vi "Maps-Update.vi"(0 "Google Maps Resource In":T1, 11 "error in (no error)":errorcluster) -> (4 "Google Maps Resource Out":T1, 8 "URL":string, 15 "error out":errorcluster)   [LabVIEW 2020]
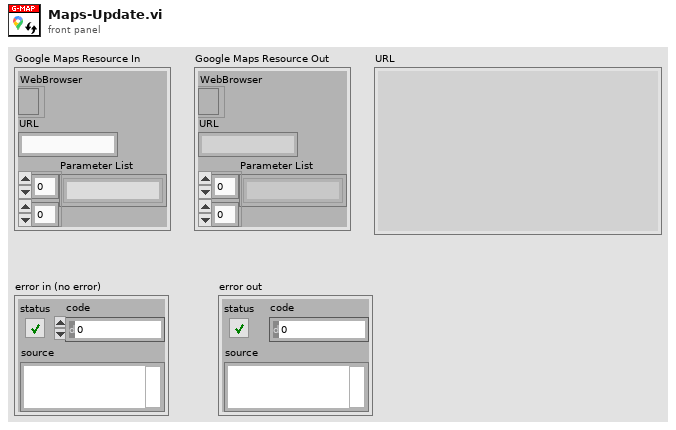
[diagram p1: front panel]
types:
  T1 = cluster{"WebBrowser":refnum<k7>, "URL":string, "Parameter List":string[][]}
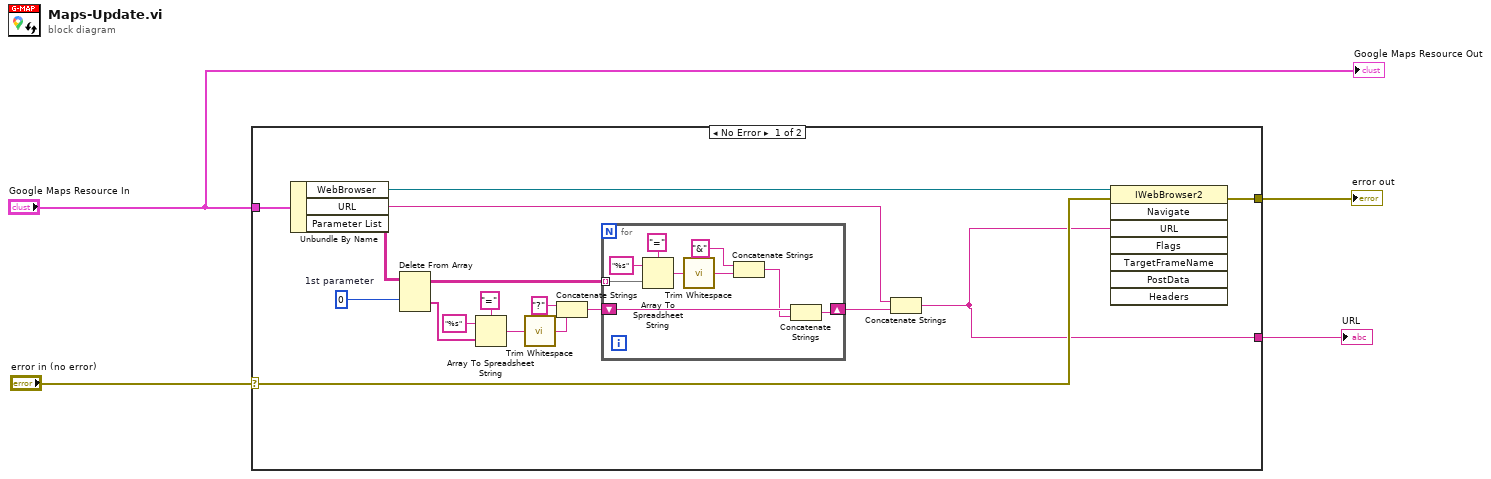
[diagram p0: block diagram]
diagram:
  n1 = case shown="No Error" "error in (no error)" {
    selector: "error in (no error)" -> [w8 w31]
    tunnel: "Google Maps Resource In" -> [w21 _]
    tunnel: [w6 w31] -> w3
    tunnel: [w5 _] -> w4
    frame No Error {
      w13 = 0  # 1st parameter
      n2 = Unbundle By Name(w21) -> ("WebBrowser"=w7:refnum<k7>, "URL"=w10:string, "Parameter List"=w20:string[][])
      n3 = Delete From Array(array=w20, index (row)=w13) -> (deleted portion=w19:string[], array with subset deleted=w12:string[][])  [unwired: 2 in]
      n4 = Array To Spreadsheet String(delimiter (Tab)="=", array=w19, 3:"%s" ("format string")) -> (spreadsheet string=w17:string)
      n5 = call <vilib>:"Trim Whitespace.vi"("string"=w17) -> ("trimmed string"=w16:string)  [unwired: 1 in]
      n6 = Concatenate Strings("?" ("string"), w16) -> (w14:string)
      n7 = for {
        shift-right: [w23] -> w11
        shift-left: w14 -> [w25]
        tunnel: w12 -> [w26] mode=indexing
        n8 = Array To Spreadsheet String(delimiter (Tab)="=", array=w26, 3:"%s" ("format string")) -> (spreadsheet string=w28:string)
        n9 = call <vilib>:"Trim Whitespace.vi"("string"=w28) -> ("trimmed string"=w29:string)  [unwired: 1 in]
        n10 = Concatenate Strings("&" ("string"), w29) -> (w24:string)
        n11 = Concatenate Strings(w25, w24) -> (w23:string)
      }
      n12 = Concatenate Strings(w10, w11) -> (w5:string)
      n13 = invoke class="IWebBrowser2" method="Navigate"(reference=w7, error in=w8, "URL"=w5) -> (error out=w6:errorcluster)  [unwired: 5 in, 7 out]
    }
    frame Error {
    }
  }
  "URL" <- w4
  "error out" <- w3
  "Google Maps Resource Out" <- "Google Maps Resource In"
